vi "Senden_ECD.vi"(5 "error in":errorcluster, 6 "BefehlsCluster":T1, 7 "AbfragenCluster":cluster{string[], string[], string[]}, 8 "Abfragenr.Cluster":cluster{i32, i32, i32}, 9 "Senden?":bool[](array[boolean]), 10 "FPGA-VI-Referenz (Ausgang)":refnum<k20>) -> (0 "BefehlsCluster":T1, 2 "error out":errorcluster, 3 "Senden?":bool[](array[boolean]), 4 "Abfragenr.Cluster":cluster{i32, i32, i32})   [LabVIEW 2017]
uses:
  GVZwischenspeicher.vi
  <vilib>/Utility/error.llb/Error Cluster From Error Code.vi
  <vilib>/rvi/errors/niLvFpgaAdjustHostInterfaceError.vi
  <vilib>/rvi/interface/nirviMethod/nirviMethod.xnode
  FPGA Bitfiles/HAGAR-V_FPGATargetECD_FPGA-ProgrammECD_LbBtUh8SPQY.lvbitx
  FPGA_ECD/FPGA-Programm_ECD.vi
  <vilib>/rvi/errors/niLvFpgaMergeErrorWithErrorCode.vi
  <vilib>/FPGAPlugInAG/cRIO-9035/niLvFpga_WriteFifo_cRIO-9035.vi
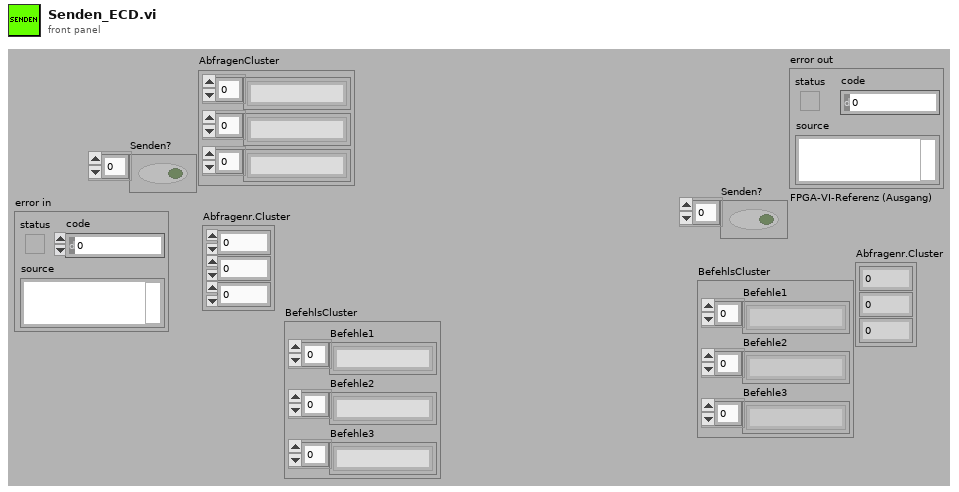
[diagram p1: front panel]
types:
  T1 = cluster{"Befehle1":string[], "Befehle2":string[], "Befehle3":string[]}
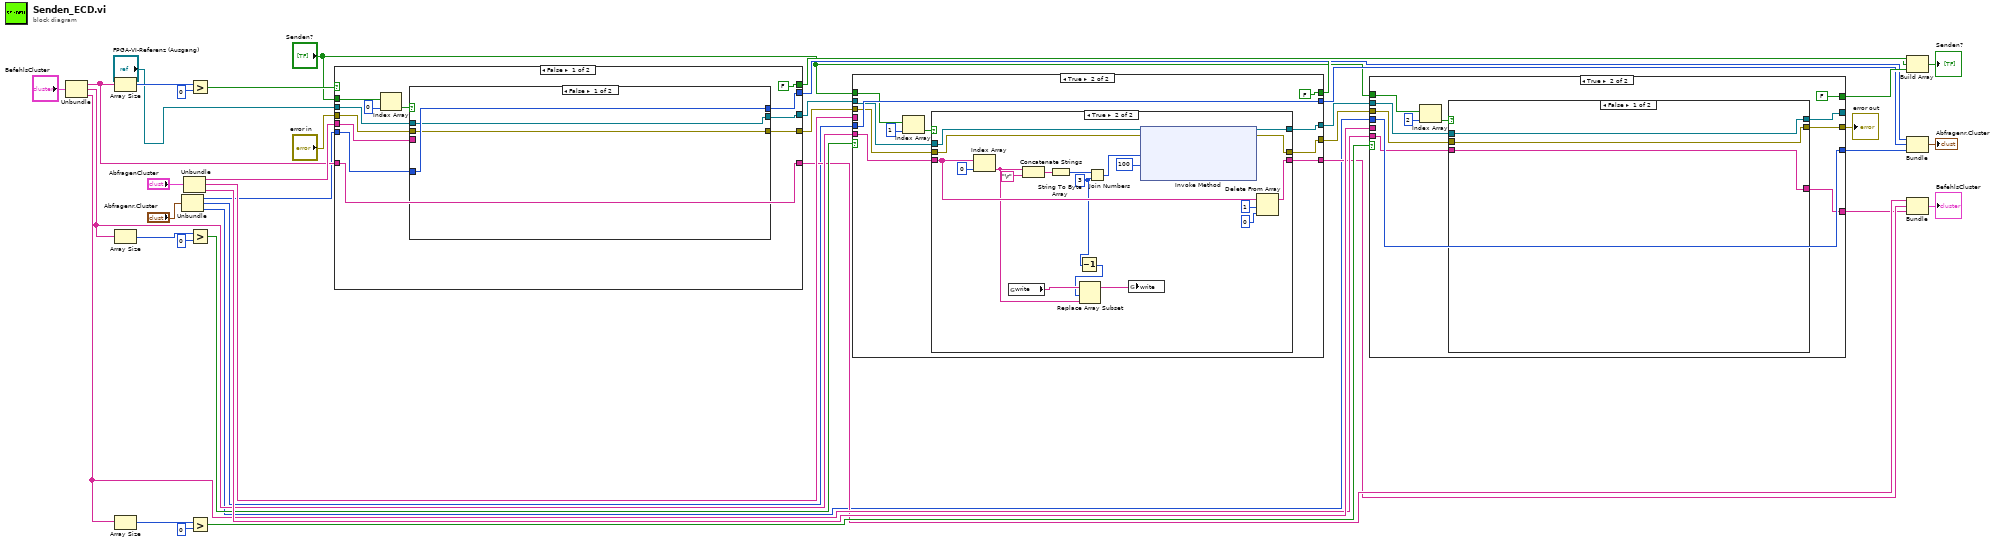
[diagram p0: block diagram]
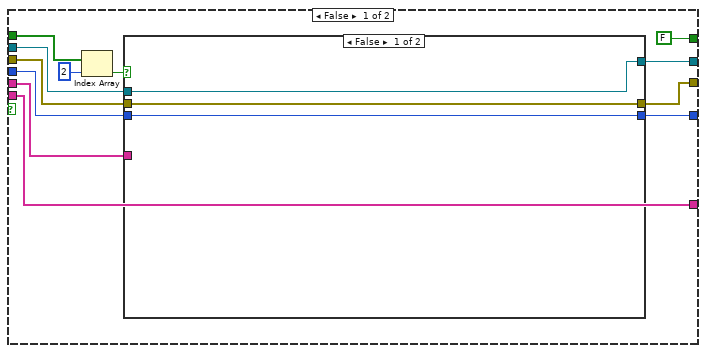
[diagram p2: hidden frame]
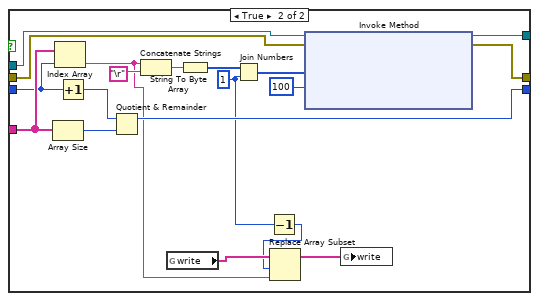
[diagram p3: hidden frame]
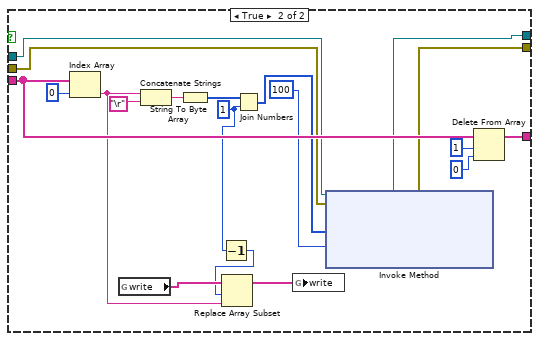
[diagram p4: hidden frame]
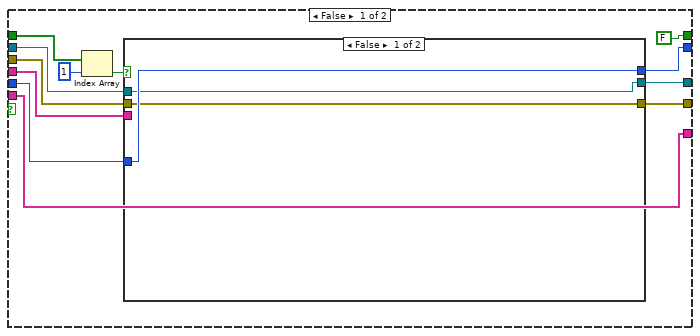
[diagram p5: hidden frame]
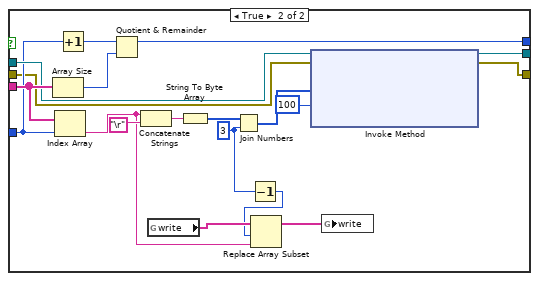
[diagram p6: hidden frame]
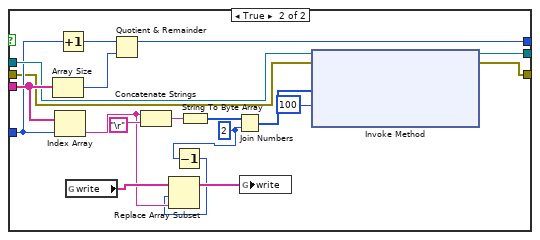
[diagram p8: hidden frame]
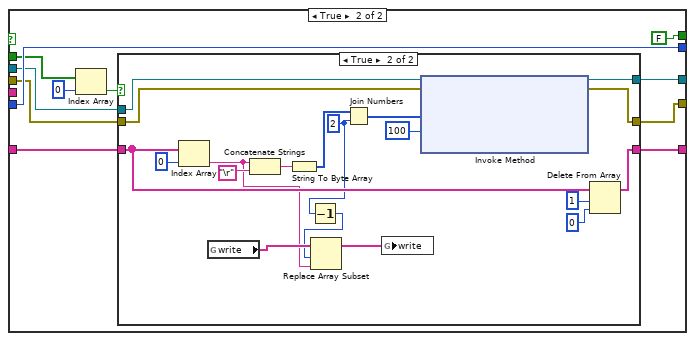
[diagram p9: hidden frame]
diagram:
  n1 = Unbundle("BefehlsCluster") -> ("Befehle1"=w26:string[], "Befehle2"=w25:string[], "Befehle3"=w24:string[])
  n2 = Array Size(array=w26) -> (size(s)=w41:i32)
  n3 = Array Size(array=w25) -> (size(s)=w35:i32)
  n4 = Array Size(array=w24) -> (size(s)=w32:i32)
  n5 = Unbundle("Abfragenr.Cluster") -> (w14:i32, w13:i32, w12:i32)
  n6 = Unbundle("AbfragenCluster") -> (w38:string[], w37:string[], w36:string[])
  n7 = Greater?(x=w41, y=0) -> (0:w39:bool)
  n8 = Greater?(x=w35, y=0) -> (0:w33:bool)
  n9 = Greater?(x=w32, y=0) -> (0:w30:bool)
  n10 = case shown="False" w39 {
    tunnel: w26 -> [w53 w83]
    tunnel: [w53 w82] -> w23
    tunnel: "Senden?" -> [w47 w80]
    tunnel: [FALSE FALSE] -> w19
    tunnel: w14 -> [w50 w86]
    tunnel: "FPGA-VI-Referenz (Ausgang)" -> [w49 w81]
    tunnel: [w48 w86] -> w11
    tunnel: w38 -> [w46 _]
    tunnel: [w45 w79] -> w29
    tunnel: "error in" -> [w43 w77]
    tunnel: [w42 w76] -> w4
    frame False {
      n11 = Index Array(array=w47, index=0 ("Index")) -> (element=w51:bool)
      n12 = case shown="False" w51 {
        tunnel: w46 -> [_ w73]
        tunnel: w50 -> [w56 w68]
        tunnel: w49 -> [w55 w71]
        tunnel: [w56 w67] -> w48
        tunnel: [w55 w66] -> w45
        tunnel: w43 -> [w54 w63]
        tunnel: [w54 w62] -> w42
        frame False {
        }
        frame True {
          w58 = u8 2
          n13 = Array Size(array=w73) -> (size(s)=w74:i32)
          n14 = Index Array(array=w73, index=w68) -> (element=w60:string)
          n15 = Increment(x=w68) -> (x+1=w75:i32)
          n16 = global read "GVZwischenspeicher.vi" "write"() -> (w61:string[])
          n17 = Quotient & Remainder(x=w75, y=w74) -> (x-y*floor(x/y)=w67:i32)  [unwired: 1 out]
          n18 = Concatenate Strings(w60, "\r") -> (w65:string)
          n19 = Decrement(x=w58) -> (x-1=w57:u8)
          n20 = Replace Array Subset(array=w61, new element=w60, index=w57) -> (w59:string[])
          n21 = String To Byte Array(string=w65) -> (unsigned byte array=w72:u8[])
          n22 = Join Numbers(hi=w72, lo=w58) -> ((hi.lo)=w70:u16[])
          n23 = global write "GVZwischenspeicher.vi" "write"(w59) -> ()
          n24 = xnode "Invoke Method"("FPGA-VI-Referenz (Eingang)"=w71, "Fehler (Eingang)"=w63, "Daten"=w70, "Timeout (ms)"=100) -> ("FPGA-VI-Referenz (Ausgang)"=w66:refnum<k20>, "Fehler (Ausgang)"=w62:errorcluster)  [unwired: 1 out]
        }
      }
    }
    frame True {
      n25 = Index Array(array=w80, index=0 ("Index")) -> (element=w84:bool)
      n26 = case shown="True" w84 {
        tunnel: w83 -> [w89 w104]
        tunnel: [w89 w106] -> w82
        tunnel: w81 -> [w88 w105]
        tunnel: [w88 w99] -> w79
        tunnel: w77 -> [w87 w96]
        tunnel: [w87 w95] -> w76
        frame False {
        }
        frame True {
          w91 = u8 2
          n27 = Index Array(array=w104, index=0 ("Index")) -> (element=w92:string)
          n28 = global read "GVZwischenspeicher.vi" "write"() -> (w94:string[])
          n29 = Concatenate Strings(w92, "\r") -> (w97:string)
          n30 = String To Byte Array(string=w97) -> (unsigned byte array=w102:u8[])
          n31 = Decrement(x=w91) -> (x-1=w90:u8)
          n32 = Replace Array Subset(array=w94, new element=w92, index=w90) -> (w93:string[])
          n33 = Join Numbers(hi=w102, lo=w91) -> ((hi.lo)=w101:u16[])
          n34 = global write "GVZwischenspeicher.vi" "write"(w93) -> ()
          n35 = xnode "Invoke Method"("FPGA-VI-Referenz (Eingang)"=w105, "Fehler (Eingang)"=w96, "Daten"=w101, "Timeout (ms)"=100) -> ("FPGA-VI-Referenz (Ausgang)"=w99:refnum<k20>, "Fehler (Ausgang)"=w95:errorcluster)  [unwired: 1 out]
          n36 = Delete From Array(array=w104, length=1 ("Länge"), index=0 ("Index")) -> (array with subset deleted=w106:string[])  [unwired: 1 out]
        }
      }
    }
  }
  n37 = case shown="True" w33 {
    tunnel: w25 -> [w120 w150]
    tunnel: [w120 w149] -> w22
    tunnel: "Senden?" -> [w114 w147]
    tunnel: w13 -> [w117 w153]
    tunnel: w29 -> [w116 w148]
    tunnel: [w115 w153] -> w10
    tunnel: w37 -> [w113 _]
    tunnel: [w112 w146] -> w28
    tunnel: [FALSE FALSE] -> w17
    tunnel: w4 -> [w110 w144]
    tunnel: [w109 w143] -> w3
    frame False {
      n38 = Index Array(array=w114, index=1 ("Index")) -> (element=w118:bool)
      n39 = case shown="False" w118 {
        tunnel: w113 -> [_ w140]
        tunnel: w117 -> [w123 w135]
        tunnel: w116 -> [w122 w138]
        tunnel: [w123 w134] -> w115
        tunnel: [w122 w133] -> w112
        tunnel: w110 -> [w121 w130]
        tunnel: [w121 w129] -> w109
        frame False {
        }
        frame True {
          w124 = u8 3
          n40 = Array Size(array=w140) -> (size(s)=w141:i32)
          n41 = Index Array(array=w140, index=w135) -> (element=w125:string)
          n42 = Increment(x=w135) -> (x+1=w142:i32)
          n43 = Quotient & Remainder(x=w142, y=w141) -> (x-y*floor(x/y)=w134:i32)  [unwired: 1 out]
          n44 = Concatenate Strings(w125, "\r") -> (w131:string)
          n45 = global read "GVZwischenspeicher.vi" "write"() -> (w128:string[])
          n46 = String To Byte Array(string=w131) -> (unsigned byte array=w139:u8[])
          n47 = Join Numbers(hi=w139, lo=w124) -> ((hi.lo)=w137:u16[])
          n48 = Decrement(x=w124) -> (x-1=w126:u8)
          n49 = Replace Array Subset(array=w128, new element=w125, index=w126) -> (w127:string[])
          n50 = xnode "Invoke Method"("FPGA-VI-Referenz (Eingang)"=w138, "Fehler (Eingang)"=w130, "Daten"=w137, "Timeout (ms)"=100) -> ("FPGA-VI-Referenz (Ausgang)"=w133:refnum<k20>, "Fehler (Ausgang)"=w129:errorcluster)  [unwired: 1 out]
          n51 = global write "GVZwischenspeicher.vi" "write"(w127) -> ()
        }
      }
    }
    frame True {
      n52 = Index Array(array=w147, index=1 ("Index")) -> (element=w151:bool)
      n53 = case shown="True" w151 {
        tunnel: w150 -> [w156 w171]
        tunnel: [w156 w173] -> w149
        tunnel: w148 -> [w155 w172]
        tunnel: [w155 w166] -> w146
        tunnel: w144 -> [w154 w163]
        tunnel: [w154 w162] -> w143
        frame False {
        }
        frame True {
          w157 = u8 3
          n54 = Index Array(array=w171, index=0 ("Index")) -> (element=w158:string)
          n55 = global read "GVZwischenspeicher.vi" "write"() -> (w161:string[])
          n56 = Concatenate Strings(w158, "\r") -> (w164:string)
          n57 = String To Byte Array(string=w164) -> (unsigned byte array=w169:u8[])
          n58 = Decrement(x=w157) -> (x-1=w159:u8)
          n59 = Replace Array Subset(array=w161, new element=w158, index=w159) -> (w160:string[])
          n60 = Join Numbers(hi=w169, lo=w157) -> ((hi.lo)=w168:u16[])
          n61 = global write "GVZwischenspeicher.vi" "write"(w160) -> ()
          n62 = xnode "Invoke Method"("FPGA-VI-Referenz (Eingang)"=w172, "Fehler (Eingang)"=w163, "Daten"=w168, "Timeout (ms)"=100) -> ("FPGA-VI-Referenz (Ausgang)"=w166:refnum<k20>, "Fehler (Ausgang)"=w162:errorcluster)  [unwired: 1 out]
          n63 = Delete From Array(array=w171, length=1 ("Länge"), index=0 ("Index")) -> (array with subset deleted=w173:string[])  [unwired: 1 out]
        }
      }
    }
  }
  n64 = case shown="True" w30 {
    tunnel: w24 -> [w187 w217]
    tunnel: [w187 w216] -> w21
    tunnel: "Senden?" -> [w181 w214]
    tunnel: w12 -> [w184 w220]
    tunnel: w28 -> [w183 w215]
    tunnel: [w182 w220] -> w9
    tunnel: w36 -> [w180 _]
    tunnel: [FALSE FALSE] -> w16
    tunnel: [w178 w212] -> _
    tunnel: w3 -> [w177 w211]
    tunnel: [w176 w210] -> w2
    frame False {
      n65 = Index Array(array=w181, index=2 ("Index")) -> (element=w185:bool)
      n66 = case shown="False" w185 {
        tunnel: w180 -> [_ w207]
        tunnel: w184 -> [w190 w202]
        tunnel: w183 -> [w189 w205]
        tunnel: [w190 w201] -> w182
        tunnel: [w189 w200] -> w178
        tunnel: w177 -> [w188 w197]
        tunnel: [w188 w196] -> w176
        frame False {
        }
        frame True {
          w191 = u8 1
          n67 = Array Size(array=w207) -> (size(s)=w208:i32)
          n68 = Index Array(array=w207, index=w202) -> (element=w192:string)
          n69 = Increment(x=w202) -> (x+1=w209:i32)
          n70 = Quotient & Remainder(x=w209, y=w208) -> (x-y*floor(x/y)=w201:i32)  [unwired: 1 out]
          n71 = Concatenate Strings(w192, "\r") -> (w198:string)
          n72 = global read "GVZwischenspeicher.vi" "write"() -> (w195:string[])
          n73 = String To Byte Array(string=w198) -> (unsigned byte array=w206:u8[])
          n74 = Join Numbers(hi=w206, lo=w191) -> ((hi.lo)=w204:u16[])
          n75 = Decrement(x=w191) -> (x-1=w193:u8)
          n76 = Replace Array Subset(array=w195, new element=w192, index=w193) -> (w194:string[])
          n77 = xnode "Invoke Method"("FPGA-VI-Referenz (Eingang)"=w205, "Fehler (Eingang)"=w197, "Daten"=w204, "Timeout (ms)"=100) -> ("FPGA-VI-Referenz (Ausgang)"=w200:refnum<k20>, "Fehler (Ausgang)"=w196:errorcluster)  [unwired: 1 out]
          n78 = global write "GVZwischenspeicher.vi" "write"(w194) -> ()
        }
      }
    }
    frame True {
      n79 = Index Array(array=w214, index=2 ("Index")) -> (element=w218:bool)
      n80 = case shown="False" w218 {
        tunnel: w217 -> [w223 w239]
        tunnel: [w223 w240] -> w216
        tunnel: w215 -> [w222 w229]
        tunnel: [w222 w227] -> w212
        tunnel: w211 -> [w221 w228]
        tunnel: [w221 w226] -> w210
        frame False {
        }
        frame True {
          w230 = u8 1
          n81 = Index Array(array=w239, index=0 ("Index")) -> (element=w231:string)
          n82 = global read "GVZwischenspeicher.vi" "write"() -> (w234:string[])
          n83 = Concatenate Strings(w231, "\r") -> (w235:string)
          n84 = String To Byte Array(string=w235) -> (unsigned byte array=w237:u8[])
          n85 = Decrement(x=w230) -> (x-1=w232:u8)
          n86 = Replace Array Subset(array=w234, new element=w231, index=w232) -> (w233:string[])
          n87 = Join Numbers(hi=w237, lo=w230) -> ((hi.lo)=w225:u16[])
          n88 = global write "GVZwischenspeicher.vi" "write"(w233) -> ()
          n89 = xnode "Invoke Method"("FPGA-VI-Referenz (Eingang)"=w229, "Fehler (Eingang)"=w228, "Daten"=w225, "Timeout (ms)"=100) -> ("FPGA-VI-Referenz (Ausgang)"=w227:refnum<k20>, "Fehler (Ausgang)"=w226:errorcluster)  [unwired: 1 out]
          n90 = Delete From Array(array=w239, length=1 ("Länge"), index=0 ("Index")) -> (array with subset deleted=w240:string[])  [unwired: 1 out]
        }
      }
    }
  }
  "error out" <- w2
  n91 = Build Array(w19, w17, w16) -> (→"Senden?":bool[])
  n92 = Bundle(w11, w10, w9) -> (→"Abfragenr.Cluster":cluster{i32, i32, i32})  [unwired: 1 in]
  n93 = Bundle("Befehle1"=w23, "Befehle2"=w22, "Befehle3"=w21) -> (→"BefehlsCluster":T1)  [unwired: 1 in]
